vi "3GradeAverageVIMarcoGonzalez.vi"() -> ()   [LabVIEW 2012]
panel:
  in  "?":bool
  out "Range":dbl(knob) scale=0.0..100.0
  in  "z":dbl
  in  "y":dbl
  in  "x":dbl
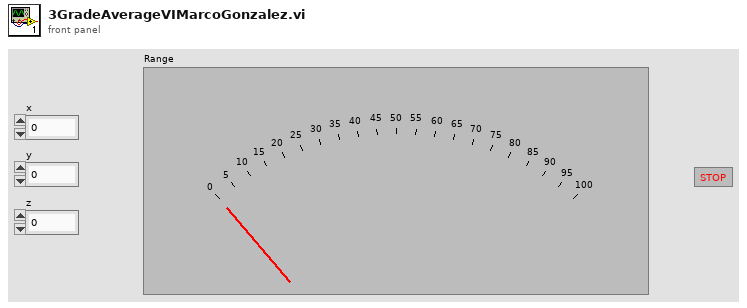
[diagram p1: front panel]
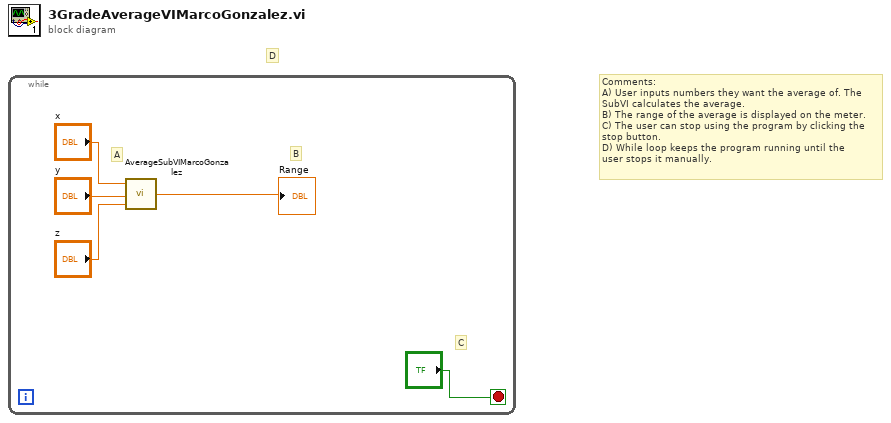
[diagram p0: block diagram]
diagram:
  # "D"
  # "Comments:\nA) User inputs numbers they want the average of. The \nSubVI calculates the average.\nB) The range of the average is displayed on the meter.\nC) The user can stop using the program by clicking the\nstop button.\nD) While loop keeps the program running until the\nuser stops it manually."
  n1 = while {
    stop <- "?" stop-if-true
    # "C"
    # "B"
    # "A"
    n2 = call "AverageSubVIMarcoGonzalez.vi"("z"="z", "y"="y", "x"="x") -> ("A"=→"Range":dbl)
  }
